vi "Day 15.vi"() -> ()   [LabVIEW 2021]
uses:
  Day 15-Position.ctl
  <vilib>/Utility/file.llb/Read Delimited Spreadsheet (string).vi
panel:
  out "Path":T1[](array[typedef])
  in  "Part 2?":bool=TRUE
  out "Min Risk":i32
  out "Input":i32[][](array[numeric])
  in  "Input File":enum32{"example input", "input"}(radio)
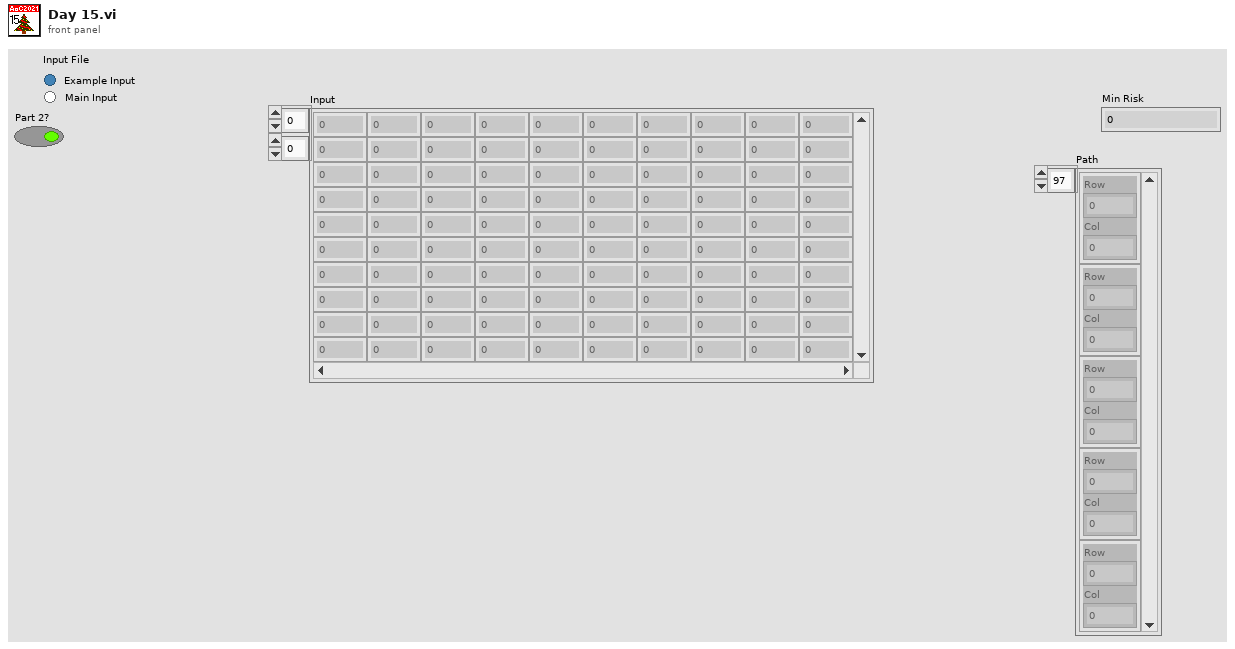
[diagram p1: front panel]
types:
  T1 = typedef "Day 15-Position.ctl" = cluster{"Row":i32, "Col":i32}
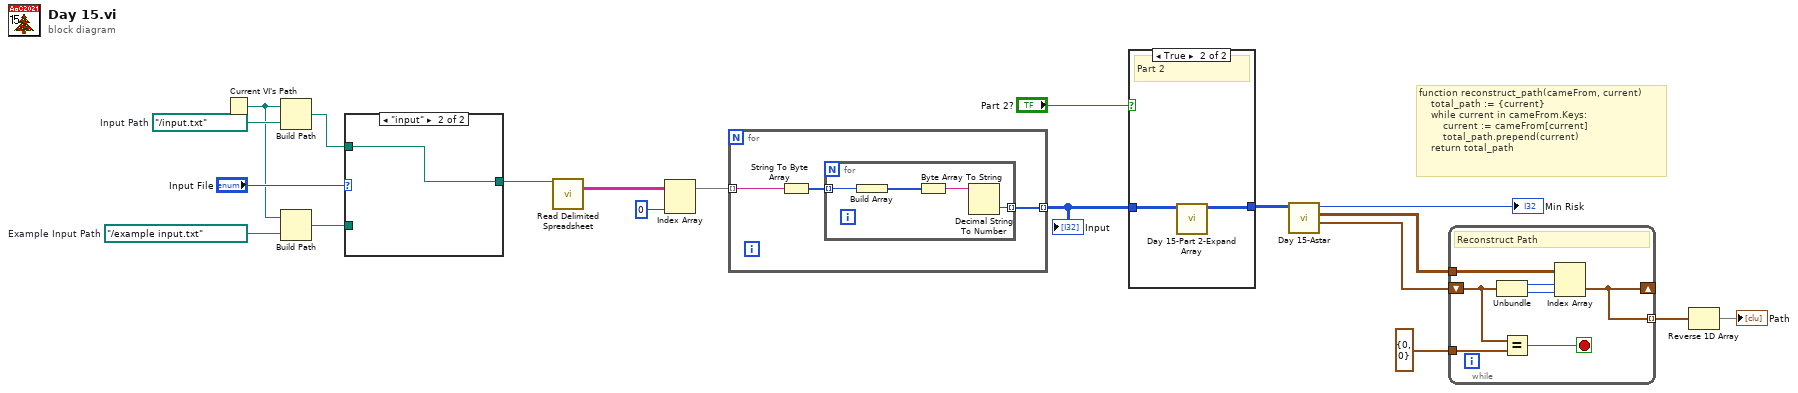
[diagram p0: block diagram]
diagram:
  w18 = path "../example input.txt"  # Example Input Path
  w19 = path "../input.txt"  # Input Path
  # "function reconstruct_path(cameFrom, current)\n    total_path := {current}\n    while current in cameFrom.Keys:\n        current := cameFrom[current]\n        total_path.prepend(current)\n    return total_path"
  n1 = Current VI's Path() -> (path=w13:path)
  n2 = Build Path(base path=w13, name or relative path=w19) -> (appended path=w16:path)
  n3 = Build Path(base path=w13, name or relative path=w18) -> (appended path=w15:path)
  n4 = case shown="\"input\"" "Input File" {
    tunnel: w16 -> [_ w21]
    tunnel: w15 -> [w20 _]
    tunnel: [w20 w21] -> w14
    frame "example input" {
    }
    frame "input" {
    }
  }
  n5 = call-poly <vilib>:"Read Delimited Spreadsheet.vi"("file path (dialog if empty)"=w14) -> ("all rows"=w12:string[][])  [unwired: 9 in, 5 out]
  n6 = Index Array(array=w12, index (col)=0 ("disabled index (col)")) -> (element=w11:string[])  [unwired: 1 in]
  n7 = for {
    tunnel: w11 -> [w24] mode=indexing
    tunnel: [w22] -> w8 mode=indexing
    n8 = String To Byte Array(string=w24) -> (unsigned byte array=w23:u8[])
    n9 = for {
      tunnel: w23 -> [w28] mode=indexing
      tunnel: [w25] -> w22 mode=indexing
      n10 = Build Array(w28) -> (w27:u8[])
      n11 = Byte Array To String(unsigned byte array=w27) -> (string=w26:string)
      n12 = Decimal String To Number(string=w26) -> (number=w25:i32)  [unwired: 2 in, 1 out]
    }
  }
  "Input" <- w8
  n13 = case shown="True" "Part 2?" {
    tunnel: w8 -> [w29 w31]
    tunnel: [w29 w30] -> w2
    frame False {
    }
    frame True {
      # "Part 2"
      n14 = call "Day 15-Part 2-Expand Array.vi"("Array in"=w31) -> ("Array out"=w30:i32[][])  [unwired: 10 in]
    }
  }
  n15 = call "Day 15-Astar.vi"("Risk[n]"=w2) -> ("Goal"=w1:T1, "cameFrom[n]"=w5:T1[][], "Minimum Risk Total"=→"Min Risk":i32)  [unwired: 8 in]
  n16 = while {
    tunnel: T1 {"Row"=0, "Col"=0} ("Position") -> [w36]
    tunnel: w5 -> [w38]
    shift-right: [w37] -> _
    shift-left: w1 -> [w32]
    tunnel: [w37] -> w4 mode=indexing
    stop <- w35 stop-if-true
    # "Reconstruct Path"
    n17 = Unbundle(w32) -> ("Row"=w34:i32, "Col"=w33:i32)
    n18 = Equal?(x=w32, y=w36) -> (x = y?=w35:bool)
    n19 = Index Array(array=w38, index (row)=w34, index (col)=w33) -> (element=w37:T1)
  }
  n20 = Reverse 1D Array(array=w4) -> (reversed array=→"Path":T1[])
